vi "Average_Of_3 subVI.vi"(1 "Variable 3":dbl, 2 "Variable 2":dbl, 3 "Variable 1":dbl) -> (0 "Mean of\nVariables":dbl)   [LabVIEW 2019]
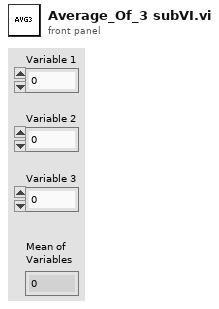
[diagram p1: front panel]
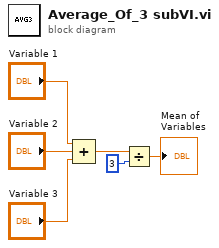
[diagram p0: block diagram]
diagram:
  n1 = Compound Arithmetic op=ADD("Variable 1", "Variable 2", "Variable 3") -> (w4:dbl)
  n2 = Divide(x=w4, y=3) -> (x/y=→"Mean of\nVariables":dbl)
